vi "Read Already Running.vi"(11 "JQMHStartup in":refnum<class "RQMHStartup.lvclass">) -> (2 "Already Running":bool, 3 "JQMHStartup out":refnum<class "RQMHStartup.lvclass">)   [LabVIEW 2024, in "RQMHStartup.lvclass"]
uses:
  RQMHStartup.lvclass
  RQMHStartup.lvclass/RQMHStartup.ctl
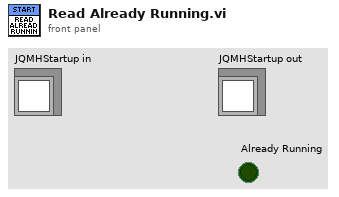
[diagram p1: front panel]
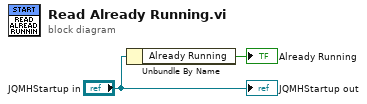
[diagram p0: block diagram]
diagram:
  n1 = Unbundle By Name("JQMHStartup in") -> ("Already Running"=→"Already Running":bool)
  "JQMHStartup out" <- "JQMHStartup in"
